vi "Configuration.vi"(5 "Vin SMU Channel":string, 8 "error in (no error)":errorcluster, 10 "Config":T1={"Voltage Level"=2.0, "Voltage Level Range"=6.0, "Current Limit"=0.01, "Current Limit Range"=0.01} {"Current Limit Range" format="%.3p"; "Current Limit" format="%.3p"; "Voltage Level Range" format="%.5p"; "Voltage Level" format="%.5p"}, 11 "IVI Refnum in":refnum<k15>) -> (0 "error out":errorcluster, 3 "IVI Refnum out":refnum<k15>)   [LabVIEW 2021, in "SMU T9.lvlib"]
uses:
  SMU T9.lvlib
  <instrlib>/niDCPower/nidcpower.llb/niDCPower Output Function.ctl
  <instrlib>/niDCPower/nidcpower.llb/niDCPower Source Mode.ctl
  controls/Configuration.ctl
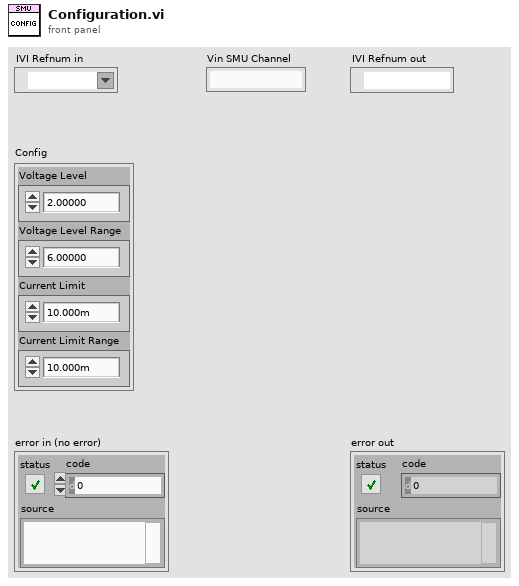
[diagram p1: front panel]
types:
  T1 = typedef "SMU T9.lvlib/Configuration.ctl" = cluster{"Voltage Level":dbl, "Voltage Level Range":dbl, "Current Limit":dbl, "Current Limit Range":dbl}
  T2 = typedef "niDCPower Output Function.ctl" = i32
  T3 = typedef "niDCPower Source Mode.ctl" = i32
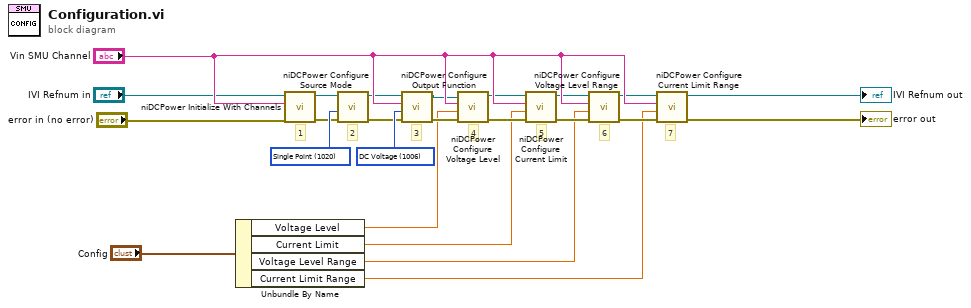
[diagram p0: block diagram]
diagram:
  w18 = T2 1006 items=["DC Voltage"=1006, "DC Current"=1007, "Pulse Voltage"=1049, "Pulse Current"=1050] ("output function")
  w11 = T3 1020 items=["Single Point"=1020, "Sequence"=1021] ("source mode")
  # "7"
  # "6"
  # "2"
  # "3"
  # "5"
  # "4"
  # "1"
  n1 = Unbundle By Name("Config") -> ("Voltage Level"=w1:dbl, "Current Limit"=w2:dbl, "Voltage Level Range"=w4:dbl, "Current Limit Range"=w3:dbl)
  n2 = call <instrlib>:"niDCPower Initialize With Channels.vi"("error in (no error)"="error in (no error)", "channels"="Vin SMU Channel", "resource name"="IVI Refnum in") -> ("error out"=w7:errorcluster, "instrument handle out"=w8:refnum<k15>)  [unwired: 2 in, 5 out]
  n3 = call <instrlib>:"niDCPower Configure Source Mode.vi"("error in (no error)"=w7, "source mode"=w11, "instrument handle"=w8) -> ("error out"=w9:errorcluster, "instrument handle out"=w10:refnum<k15>)  [unwired: 7 out]
  n4 = call <instrlib>:"niDCPower Configure Output Function.vi"("error in (no error)"=w9, "output function"=w18, "channel name"="Vin SMU Channel", "instrument handle"=w10) -> ("error out"=w17:errorcluster, "instrument handle out"=w16:refnum<k15>)  [unwired: 6 out]
  n5 = call <instrlib>:"niDCPower Configure Voltage Level.vi"("error in (no error)"=w17, "voltage level"=w1, "channel name"="Vin SMU Channel", "instrument handle"=w16) -> ("error out"=w6:errorcluster, "instrument handle out"=w5:refnum<k15>)  [unwired: 6 out]
  n6 = call <instrlib>:"niDCPower Configure Current Limit.vi"("error in (no error)"=w6, "current limit"=w2, "channel name"="Vin SMU Channel", "instrument handle"=w5) -> ("error out"=w12:errorcluster, "instrument handle out"=w13:refnum<k15>)  [unwired: 1 in, 5 out]
  n7 = call <instrlib>:"niDCPower Configure Voltage Level Range.vi"("error in (no error)"=w12, "voltage level range"=w4, "channel name"="Vin SMU Channel", "instrument handle"=w13) -> ("error out"=w14:errorcluster, "instrument handle out"=w15:refnum<k15>)  [unwired: 6 out]
  n8 = call <instrlib>:"niDCPower Configure Current Limit Range.vi"("error in (no error)"=w14, "current limit range"=w3, "channel name"="Vin SMU Channel", "instrument handle"=w15) -> ("error out"=→"error out":errorcluster, "instrument handle out"=→"IVI Refnum out":refnum<k15>)  [unwired: 6 out]
